vi "Write Center Point.vi"(10 "Center Point":dbl[unit], 11 "PressureServoCylinderActuator in":refnum<class "PressureServoCylinderActuator.lvclass">) -> (3 "PressureServoCylinderActuator out":refnum<class "PressureServoCylinderActuator.lvclass">)   [LabVIEW 2015, in "PressureServoCylinderActuator.lvclass"]
uses:
  PressureServoCylinderActuator.lvclass
  PressureServoCylinderActuator.lvclass/PressureServoCylinderActuator.ctl
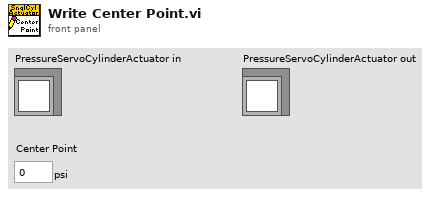
[diagram p1: front panel]
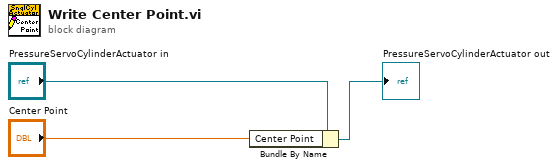
[diagram p0: block diagram]
diagram:
  n1 = Bundle By Name(cluster="PressureServoCylinderActuator in", "Center Point"="Center Point") -> (→"PressureServoCylinderActuator out":refnum<class "PressureServoCylinderActuator.lvclass">)
